vi "PH_BeamlineController.set PA DP Target Elements to be enabled.vi"(0 "VI in":refnum<vi>, 5 "error in (no error)":errorcluster) -> (14 "VI out":refnum<vi>, 19 "error out":errorcluster)   [LabVIEW 2014, in "PH_BeamlineController.lvlib"]
uses:
  PH_BeamlineController.lvlib
  PH_Beamline_Chief/PH_Beamline_Chief.Section.ctl
  PH_BeamlineInformation/PH_BeamlineInformation.lvlib
  PH_Beamline_Chief/PH_Beamline_Chief.lvlib
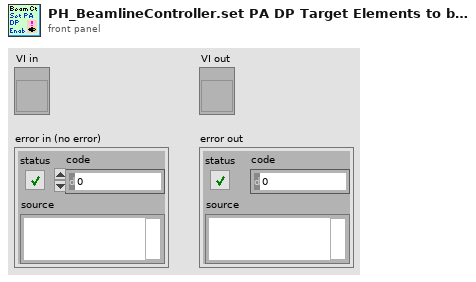
[diagram p1: front panel]
types:
  T1 = typedef "PH_Beamline_Chief.lvlib/PH_Beamline_Chief.Section.ctl" = enum16{"None", "YLF", "fs", "fs-YLF", "ns", "PA-Input", "PA-Undelay", "PA-Delay", "PA-before-Bypass", "PA", "PA-Bypass", "PA-Exit", "PA-LL", "LL", "PA-MA", "MA-Exit", "MA-Z6", "Z6", "MA-LB", "LB-TB2", "LB-TB3"}
  T2 = typedef "PH_BeamlineController.lvlib/PH_BeamlineController.i attribute.ctl" = cluster{"Vacuum Exp LB":cluster{"Channel":string, "Limit [mbar]":dbl, "Pressure [mbar]":dbl, "GUI Ref":refnum<vi>}, "Sources":T3[], "PA DP Targets":T5[], "Path":cluster{"Source":T4, "PA DP Target":T6, "Target":T7}, "Targets":cluster{"Name":T7, "GUI Ref":refnum<vi>, "Current State":bool, "Wanted State":bool, "Enabled":bool}[], "Status Tags":cluster{"Name":string, "Status":T8}[], "special GUI Refs":T9}
  T3 = typedef "PH_BeamlineController.lvlib/PH_BeamlineController.Source Attributes.ctl" = cluster{"Name":T4, "GUI Ref":refnum<vi>, "Current State":bool, "Wanted State":bool}
  T4 = typedef "PH_BeamlineController.lvlib/PH_BeamlineController.Sources.ctl" = enum16{"None", "YLF", "fs-Frontend", "ns-Frontend", "YLF and ns-Frontend", "fs- and ns-Frontend"}
  T5 = typedef "PH_BeamlineController.lvlib/PH_BeamlineController.PA DP Target Attributes.ctl" = cluster{"Name":T6, "GUI Ref":refnum<vi>, "Current State":bool, "Wanted State":bool, "Enabled":bool}
  T6 = typedef "PH_BeamlineController.lvlib/PH_BeamlineController.PA DP Targets.ctl" = enum16{"None", "Dump PA Delayed Beam", "Dump PA Undelayed Beam", "Dumps PA Delayed and Undelayed Beam"}
  T7 = typedef "PH_BeamlineController.lvlib/PH_BeamlineController.Targets.ctl" = enum16{"None", "PreAmp", "Dump Exp Laserlab", "Exp Laserlab", "Calorimeter", "Dump Exp Laserbay", "Exp Laserbay", "Dump Exp Z6", "Exp Z6"}
  T8 = typedef "PH_StatusHandler.lvlib/PH_StatusHandler.Status.ctl" = i16
  T9 = typedef "PH_BeamlineController.lvlib/PH_BeamlineController.special GUI Refs.ctl" = cluster{"PA-Backreflection-Meas":refnum<vi>, "fs_Synchrolock_Watch":refnum<vi>}
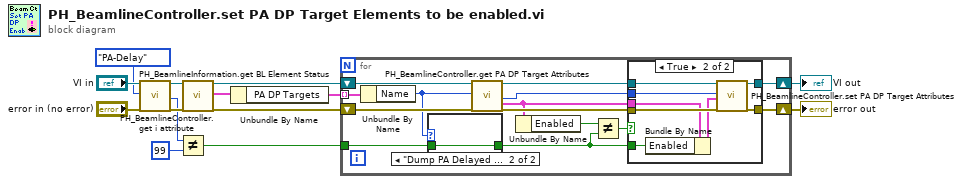
[diagram p0: block diagram]
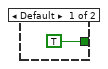
[diagram p2: hidden frame]
diagram:
  n1 = call "PH_BeamlineInformation.get BL Element Status.vi"("VI in"="VI in", "Beamline Element"=PH_Beamline_Chief.Section."PA-Delay", "error in (no error)"="error in (no error)") -> ("VI out"=w5:refnum<vi>, "Status"=w3:i32, "error out"=w7:errorcluster)  [unwired: 14 in]
  n2 = Not Equal?(x=w3, y=99 ("Status")) -> (x != y?=w1:bool)
  n3 = call "PH_BeamlineController.get i attribute.vi"("i ref in"=w5, "error in (no error)"=w7) -> ("i ref out"=w11:refnum<vi>, "i attribute"=w12:T2, "error out"=w14:errorcluster)  [unwired: 15 in]
  n4 = Unbundle By Name(w12) -> ("PA DP Targets"=w8:T5[])
  n5 = for {
    shift-right: [w25] -> w10
    shift-left: w14 -> [w28]
    shift-right: [w23] -> w9
    shift-left: w11 -> [w26]
    tunnel: w8 -> [w21] mode=indexing
    tunnel: w1 -> [w15]
    n6 = Unbundle By Name(w21) -> ("Name"=w16:T6)
    n7 = case shown="\"Dump PA Delayed Beam\", \"Dump PA Undelayed Beam\"" w16 {
      tunnel: [TRUE w30] -> w18
      tunnel: w15 -> [_ w30]
      frame Default {
      }
      frame "Dump PA Delayed Beam", "Dump PA Undelayed Beam" {
      }
    }
    n8 = call "PH_BeamlineController.get PA DP Target Attributes.vi"("VI in"=w26, "PA DP Target"=w16, "error in (no error)"=w28) -> ("VI out"=w24:refnum<vi>, "PA DP Target Index"=w22:i32, "PA DP Target Attributes"=w20:T5, "error out"=w27:errorcluster)  [unwired: 13 in]
    n9 = Unbundle By Name(w20) -> ("Enabled"=w19:bool)
    n10 = Not Equal?(x=w19, y=w18) -> (x != y?=w17:bool)
    n11 = case shown="True" w17 {
      tunnel: w27 -> [w31 w40]
      tunnel: [w31 w39] -> w25
      tunnel: w24 -> [w32 w38]
      tunnel: [w32 w37] -> w23
      tunnel: w22 -> [_ w36]
      tunnel: w20 -> [_ w34]
      tunnel: w18 -> [_ w33]
      frame False {
      }
      frame True {
        n12 = Bundle By Name(cluster=w34, "Enabled"=w33) -> (w35:T5)
        n13 = call "PH_BeamlineController.set PA DP Target Attributes.vi"("VI in"=w38, "PA DP Target Index"=w36, "Changed PA DP Target Attributes"=w35, "error in (no error)"=w40) -> ("VI out"=w37:refnum<vi>, "error out"=w39:errorcluster)  [unwired: 14 in]
      }
    }
  }
  "VI out" <- w9
  "error out" <- w10
